vi "Write Product Name - Unique Name.vi"(8 "error in (no error)":errorcluster, 10 "Product Name -> Unique Name":variant, 11 "Build Analyzer in":refnum<class "Build Analyzer.lvclass">) -> (0 "error out":errorcluster, 3 "Build Analyzer out":refnum<class "Build Analyzer.lvclass">)   [LabVIEW 2017, in "CL_G3_VIComponentBuilder.lvlib" / "Build Analyzer.lvclass"]
doc: "Writes the map (as a variant lookup table) between Product Name and unique name of the component."
uses:
  Build Analyzer.lvclass
  Build Analyzer.lvclass/Build Analyzer.ctl
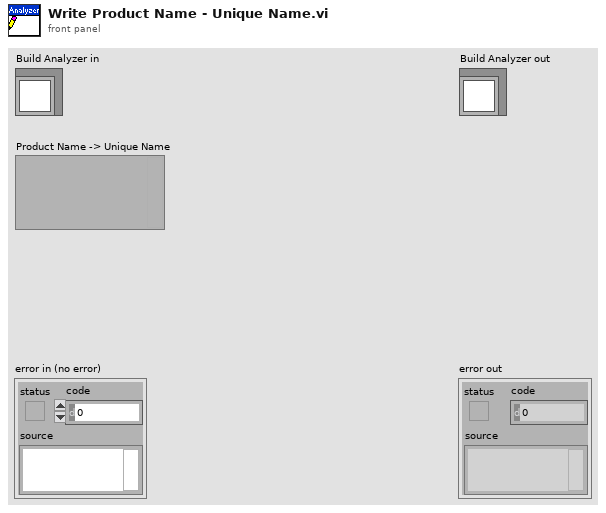
[diagram p1: front panel]
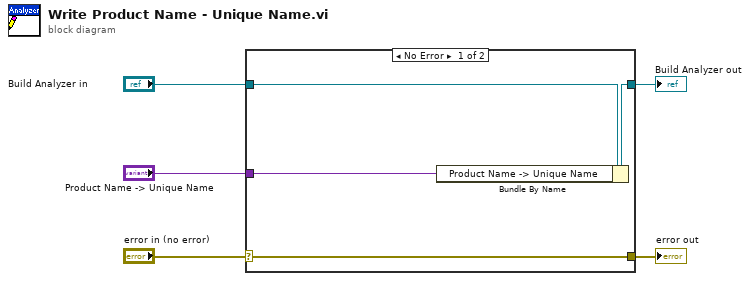
[diagram p0: block diagram]
diagram:
  n1 = case shown="No Error" "error in (no error)" {
    selector: "error in (no error)" -> [w9 w10]
    tunnel: [w9 w10] -> w4
    tunnel: [w7 w11] -> w2
    tunnel: "Build Analyzer in" -> [w8 w11]
    tunnel: "Product Name -> Unique Name" -> [w6 _]
    frame No Error {
      n2 = Bundle By Name(cluster=w8, "Product Name -> Unique Name"=w6) -> (w7:refnum<class "Build Analyzer.lvclass">)
    }
    frame Error {
    }
  }
  "error out" <- w4
  "Build Analyzer out" <- w2
